vi "Envelope.vi"(10 "L 2":dbl(slide)=85.0 scale=0.0..200.0, 11 "L 1":dbl(slide)=77.5 scale=0.0..200.0) -> (2 "new picture":picture)   [LabVIEW 2024]
panel:
  out "Array 3":cluster{dbl, dbl}[](array[cluster])
  out "Array 2":cluster{dbl, dbl}[](array[cluster])
  out "Array":cluster{dbl, dbl}[](array[cluster])
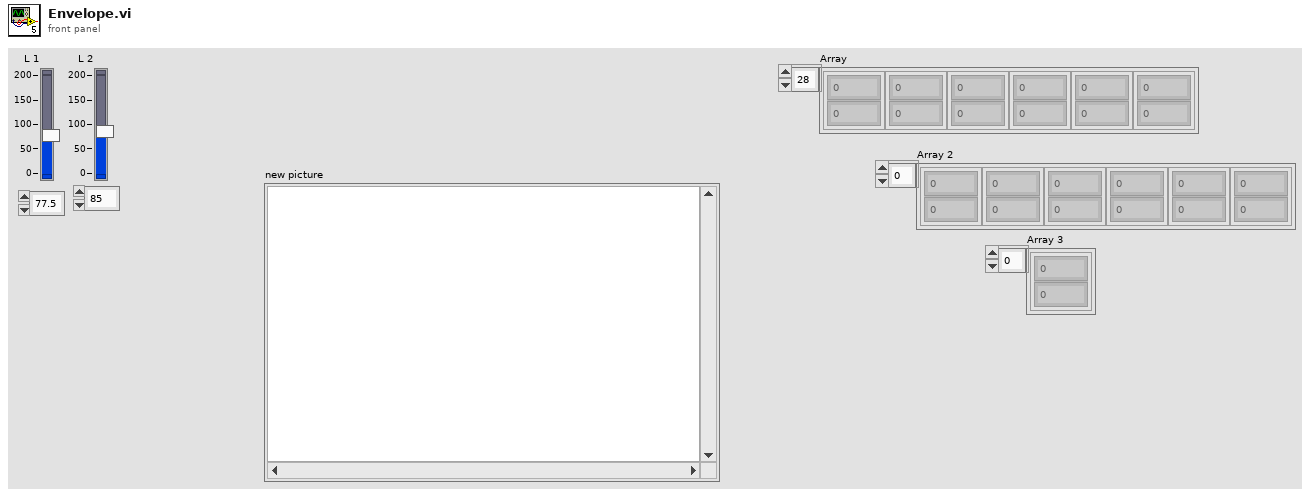
[diagram p1: front panel]
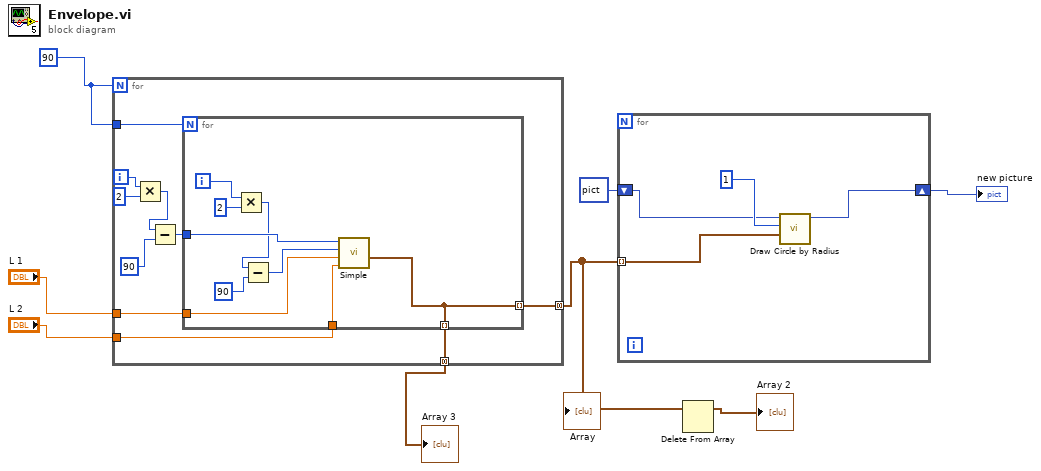
[diagram p0: block diagram]
diagram:
  w8 = 90
  n1 = for {
    N: w8 -> [_]
    tunnel: w8 -> [w18]
    tunnel: [w15] -> w2 mode=concatenating
    tunnel: "L 1" -> [w14]
    tunnel: "L 2" -> [w13]
    tunnel: [w12] -> w1 mode=concatenating
    i -> [w11]
    n2 = Multiply(x=w11, y=2) -> (x*y=w9:i32)
    n3 = Subtract(x=w9, y=90) -> (x-y=w16:i32)
    n4 = for {
      N: w18 -> [_]
      tunnel: w16 -> [w26]
      tunnel: [w22] -> w15 mode=indexing
      tunnel: w14 -> [w24]
      tunnel: w13 -> [w23]
      tunnel: [w22] -> w12 mode=indexing
      i -> [w20]
      n5 = Multiply(x=w20, y=2) -> (x*y=w19:i32)
      n6 = Subtract(x=w19, y=90) -> (x-y=w25:i32)
      n7 = call <userlib>:"Simple.vi"("L 2"=w23, "L 1"=w24, "Angle 2"=w25, "Angle1"=w26) -> ("Final 2D Pos"=w22:cluster{dbl, dbl})  [unwired: 5 in, 2 out]
    }
  }
  "Array" <- w2
  "Array 3" <- w1
  n8 = for {
    tunnel: w2 -> [w30] mode=indexing
    shift-right: [w28] -> w3
    shift-left: picture data[5B] ("new picture") -> [w29]
    n9 = call <vilib>:"Draw Circle by Radius.vi"("pixel center"=w30, "radius"=i16 1, "picture"=w29) -> ("new picture"=w28:picture)  [unwired: 8 in]
  }
  "new picture" <- w3
  n10 = Delete From Array(array=w2) -> (array with subset deleted=→"Array 2":cluster{dbl, dbl}[])  [unwired: 2 in, 1 out]
